vi "testdatabase.vi"() -> ()   [LabVIEW 2023]
uses:
  <vilib>/addons/database/Auxilliary.llb/DB Tools Cursor Type.ctl
  <vilib>/addons/database/Connection.llb/DB Tools Open Connec (Path).vi
  <vilib>/addons/database/Recordset.llb/Rec Destroy - Connection.vi
  <vilib>/addons/database/Connection.llb/Conn Execute.vi
  <vilib>/addons/database/NI_Database_API.lvlib
panel:
  out "result string":string
  in  "stop":bool
  in  "Insert":bool
  in  "Numbers":string
  in  "Names":string
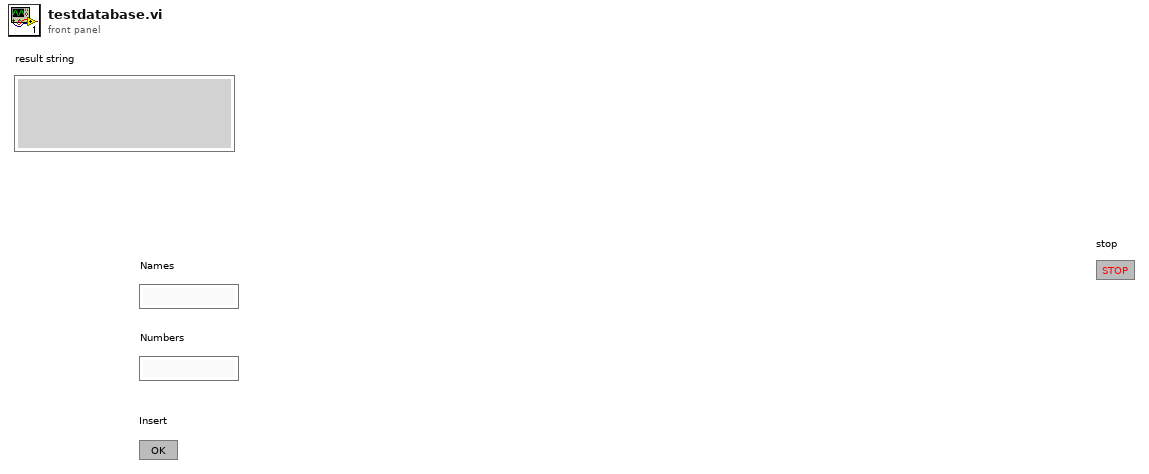
[diagram p1: front panel]
types:
  T1 = typedef "NI_Database_API.lvlib/DB Tools Cursor Type.ctl" = enum16{"forward-only", "keyset", "dynamic", "static"}
  T2 = typedef "NI_Database_API.lvlib/Conn ObjectReference.ctl" = refnum<k1>
  T3 = typedef "NI_Database_API.lvlib/Rec ObjectReference.ctl" = refnum<k1>
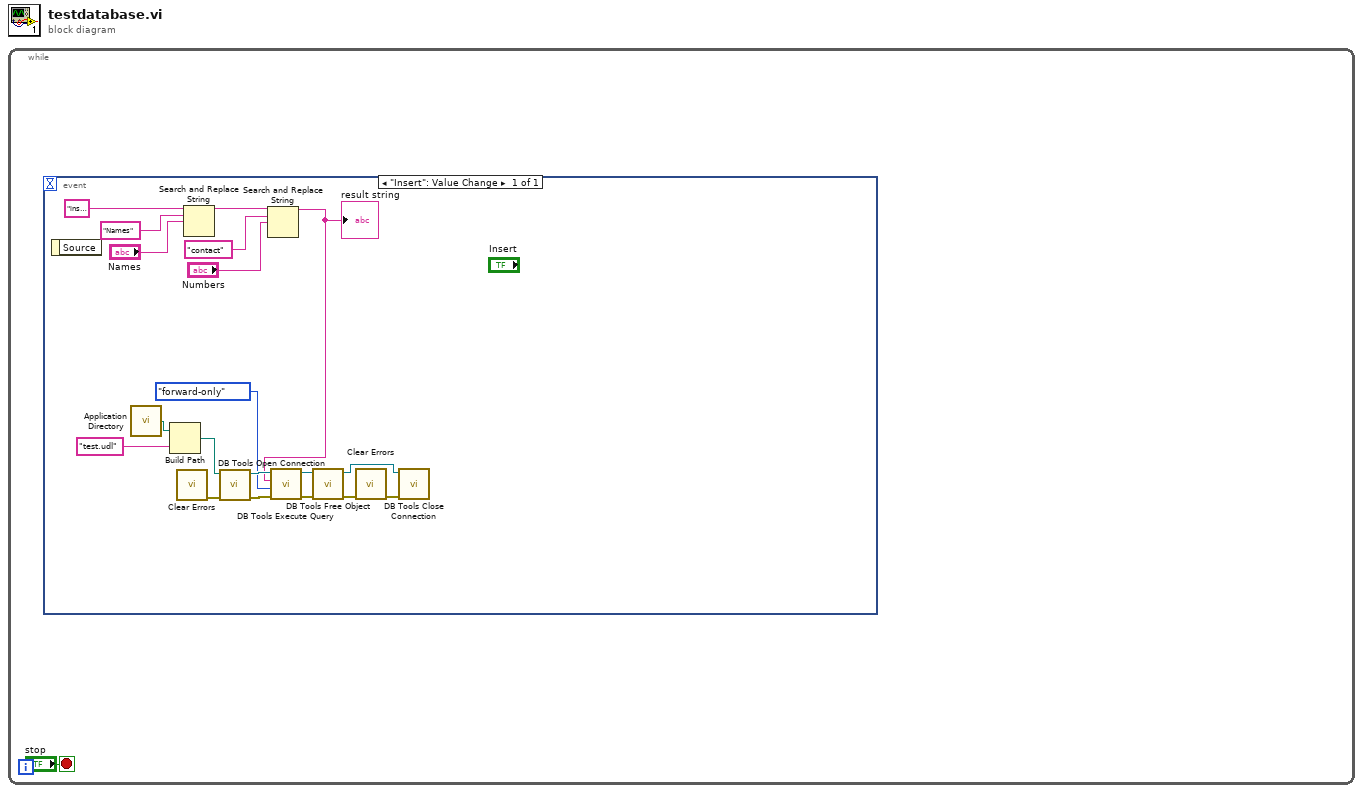
[diagram p0: block diagram]
diagram:
  n1 = while {
    stop <- "stop" stop-if-true
    n2 = event shown="[0] \"Insert\": Value Change" {
      selector: _ -> [_]
      dyn-events: _ -> [_]
      timeout: _ -> [_]
      event "Insert": Value Change {
        n3 = event-data() -> ()  [unwired: 1 in, 1 out]
        n4 = call <vilib>:"Application Directory.vi"() -> ("Application Directory"=w15:path)
        n5 = Build Path(base path=w15, name or relative path="test.udl") -> (appended path=w12:path)
        n6 = call <vilib>:"Clear Errors.vi"() -> ("error out"=w13:errorcluster)  [unwired: 6 in, 1 out]
        n7 = Search and Replace String(input string="insert into Numbers values ('Names','contact')", search string="Names", replace string="Names") -> (result string=w10:string)  [unwired: 5 in, 3 out]
        n8 = call-poly <vilib>:"DB Tools Open Connection.vi"("error in (no error)"=w13, "connection information"=w12) -> ("error out"=w19:errorcluster, "connection reference"=w20:T2)  [unwired: 6 in]
        n9 = Search and Replace String(input string=w10, search string="contact", replace string="Numbers") -> (result string=w2:string)  [unwired: 5 in, 3 out]
        "result string" <- w2
        n10 = call-poly <vilib>:"DB Tools Execute Query.vi"("error in (no error)"=w19, "cursor type"=DB_Tools_Cursor_Type."forward-only", "SQL query"=w2, "connection reference"=w20) -> ("error out"=w3:errorcluster, "recordset reference"=w4:T3)  [unwired: 4 in]
        n11 = call-poly <vilib>:"DB Tools Free Object.vi"("error in (no error)"=w3, "recordset reference"=w4) -> ("error out"=w16:errorcluster, "connection reference"=w18:T2)  [unwired: 8 in]
        n12 = call <vilib>:"Clear Errors.vi"("error in (no error)"=w16) -> ("error out"=w17:errorcluster)  [unwired: 5 in, 1 out]
        n13 = call <vilib>:"DB Tools Close Connection.vi"("error in (no error)"=w17, "connection reference"=w18) -> ()  [unwired: 5 in, 1 out]
      }
    }
  }
